vi "Cleanup all Wiring.vi"() -> ()   [LabVIEW 2012]
uses:
  Scripting Tools.lvlib
panel:
  out "Message":string
  out "Prgoress":sgl(slide) scale=0.0..1.0
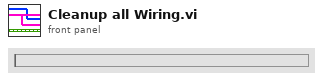
[diagram p1: front panel]
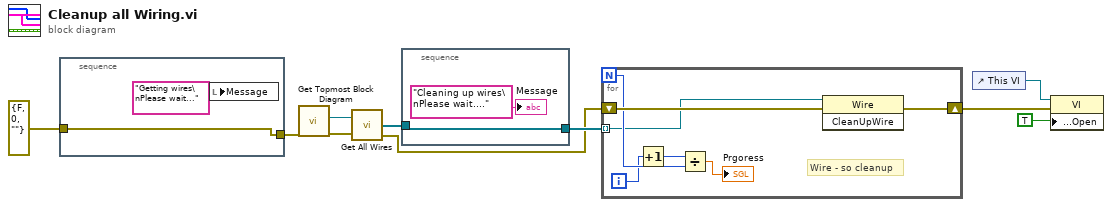
[diagram p0: block diagram]
diagram:
  n1 = stacked-sequence {
    tunnel: [w11] -> w5
    tunnel: errorcluster {"status"=FALSE, "code"=0, "source"=""} ("error in") -> [w11]
    frame #0 {
      n2 = local write "Message"("Getting wires\nPlease wait..." ("Message")) -> ()
    }
  }
  n3 = call "Get Topmost Block Diagram.vi"("error in (no error)"=w5) -> ("error out"=w4:errorcluster, "Reference to Diagram"=w3:refnum<vi>)  [unwired: 9 out]
  n4 = call "Get All Wires.vi"("Diagram In"=w3, "error in"=w4) -> ("All Wires"=w2:refnum<vi>[], "error out"=w1:errorcluster)  [unwired: 1 out]
  n5 = stacked-sequence {
    tunnel: [w13] -> w10
    tunnel: w2 -> [w13]
    frame #0 {
      "Message" <- "Cleaning up wires\nPlease wait...." ("Message")
    }
  }
  n6 = for {
    N -> [w19]
    shift-right: [w20] -> w7
    shift-left: w1 -> [w21]
    tunnel: w10 -> [w15] mode=indexing
    i -> [w18]
    # "Wire - so cleanup"
    n7 = Increment(x=w18) -> (x+1=w17:i32)
    n8 = Divide(x=w17, y=w19) -> (x/y=→"Prgoress":dbl)
    n9 = invoke class="Wire" method="CleanUpWire"(reference=w15, error in=w21) -> (error out=w20:errorcluster)  [unwired: 1 in, 2 out]
  }
  n10 = control-ref of="This VI"() -> (w8:refnum<vi>)
  n11 = property class="VI"(reference=w8, error in=w7, "Front Panel.Open"=TRUE ("Front Panel Window:Open")) -> ()  [unwired: 2 out]
